vi "facing subvi.vi"(9 "Compass":dbl, 10 "Robot Angle":dbl, 11 "Left?":bool) -> (3 "Facing":dbl)   [LabVIEW 2018]
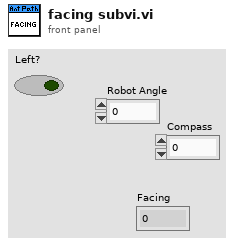
[diagram p1: front panel]
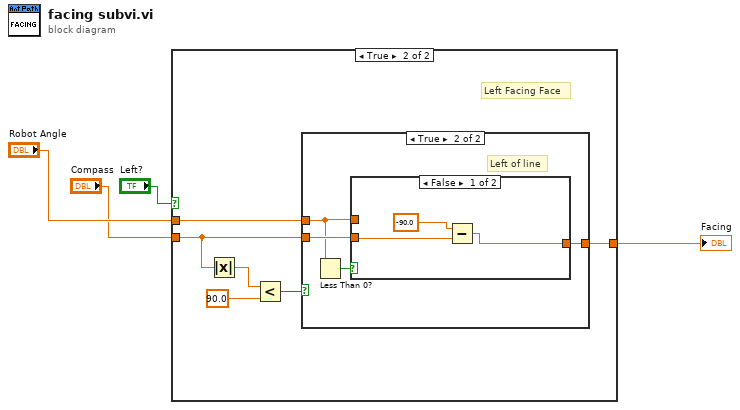
[diagram p0: block diagram]
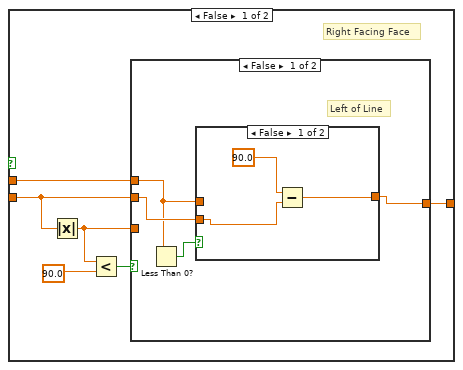
[diagram p2: hidden frame]
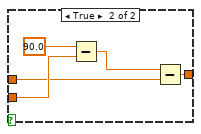
[diagram p3: hidden frame]
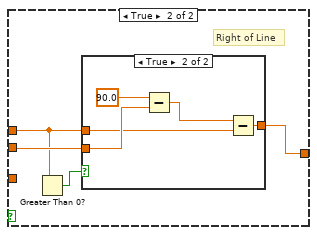
[diagram p4: hidden frame]
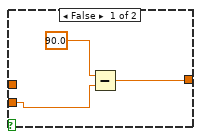
[diagram p5: hidden frame]
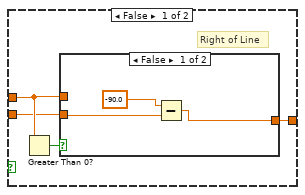
[diagram p6: hidden frame]
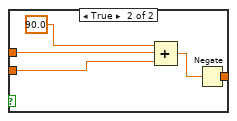
[diagram p7: hidden frame]
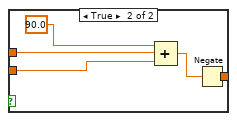
[diagram p8: hidden frame]
diagram:
  n1 = case shown="True" "Left?" {
    tunnel: "Robot Angle" -> [w8 w36]
    tunnel: "Compass" -> [w5 w35]
    tunnel: [w10 w40] -> w4
    frame False {
      # "Right Facing Face"
      n2 = Absolute Value(x=w5) -> (abs(x)=w9:dbl)
      n3 = Less?(x=w9, y=90.0) -> (x < y?=w6:bool)
      n4 = case shown="False" w6 {
        tunnel: w8 -> [w12 w24]
        tunnel: [w11 w26] -> w10
        tunnel: w9 -> [_ _]
        tunnel: w5 -> [w13 w25]
        frame False {
          # "Left of Line"
          n5 = Less Than 0?(x=w12) -> (x < 0?=w14:bool)
          n6 = case shown="False" w14 {
            tunnel: [w15 w20] -> w11
            tunnel: w13 -> [w16 w19]
            tunnel: w12 -> [_ w18]
            frame False {
              n7 = Subtract(x=90.0, y=w16) -> (x-y=w15:dbl)
            }
            frame True {
              n8 = Subtract(x=90.0, y=w19) -> (x-y=w21:dbl)
              n9 = Subtract(x=w21, y=w18) -> (x-y=w20:dbl)
            }
          }
        }
        frame True {
          # "Right of Line"
          n10 = Greater Than 0?(x=w24) -> (x > 0?=w23:bool)
          n11 = case shown="True" w23 {
            tunnel: [w27 w32] -> w26
            tunnel: w25 -> [w28 w31]
            tunnel: w24 -> [_ w30]
            frame False {
              n12 = Subtract(x=90.0, y=w28) -> (x-y=w27:dbl)
            }
            frame True {
              n13 = Subtract(x=90.0, y=w31) -> (x-y=w33:dbl)
              n14 = Subtract(x=w33, y=w30) -> (x-y=w32:dbl)
            }
          }
        }
      }
    }
    frame True {
      # "Left Facing Face"
      n15 = Absolute Value(x=w35) -> (abs(x)=w39:dbl)
      n16 = Less?(x=w39, y=90.0) -> (x < y?=w37:bool)
      n17 = case shown="True" w37 {
        tunnel: w36 -> [w43 w54]
        tunnel: w35 -> [w42 w55]
        tunnel: [w41 w56] -> w40
        frame False {
          # "Right of Line"
          n18 = Greater Than 0?(x=w43) -> (x > 0?=w44:bool)
          n19 = case shown="False" w44 {
            tunnel: [w45 w50] -> w41
            tunnel: w42 -> [w46 w49]
            tunnel: w43 -> [_ w48]
            frame False {
              n20 = Subtract(x=-90.0, y=w46) -> (x-y=w45:dbl)
            }
            frame True {
              n21 = Compound Arithmetic op=ADD(90.0, w48, w49) -> (w51:dbl)
              n22 = Negate(x=w51) -> (-x=w50:dbl)
            }
          }
        }
        frame True {
          # "Left of line"
          n23 = Less Than 0?(x=w54) -> (x < 0?=w53:bool)
          n24 = case shown="False" w53 {
            tunnel: [w57 w62] -> w56
            tunnel: w55 -> [w58 w61]
            tunnel: w54 -> [_ w60]
            frame False {
              n25 = Subtract(x=-90.0, y=w58) -> (x-y=w57:dbl)
            }
            frame True {
              n26 = Compound Arithmetic op=ADD(90.0, w60, w61) -> (w63:dbl)
              n27 = Negate(x=w63) -> (-x=w62:dbl)
            }
          }
        }
      }
    }
  }
  "Facing" <- w4
